vi "Begin.vi"(8 "error in":errorcluster) -> (0 "error out":errorcluster)   [LabVIEW 2016]
doc: "Called before other user functions, this VI is expected to open initial I/O refnums, load in file data, and do all program initialization. Notice that the <B>error out</B> terminal is simply used for data flow. Wiring it to other structures or subVIs ensures that this VI runs first."
uses:
  <vilib>/Rock Robotics/SystemInterfaces/DIO/FPGA_DIOPWMChannel.ctl
  <vilib>/Rock Robotics/WPI/SafetyOutput/WPI_SafetyOutputConfigMenu.ctl
  <vilib>/Rock Robotics/WPI/DriverStation/WPI_DriverStationRobotMode2.ctl
  <vilib>/Rock Robotics/WPI/Joystick/WPI_JoystickDeviceEnum.ctl
  <vilib>/Rock Robotics/SystemInterfaces/DIO/FPGA_DIOChannel.ctl
  <vilib>/Rock Robotics/WPI/RobotDrive/WPI_RobotDriveOpen2MotorWithVictorSP.vi
  Robot Global Data.vi
  <vilib>/Rock Robotics/Network Tables/NT Write String Array.vi
  <vilib>/Rock Robotics/WPI/MotorControl/WPI_MotorControlOpen SPARK.vi
  <vilib>/Rock Robotics/WPI/MotorControl/WPI_MotorControlOpen VictorSP.vi
  <vilib>/Rock Robotics/WPI/Counter/WPI_CounterDigitalInputToDigitalSource.vi
  <vilib>/Rock Robotics/WPI/Counter/WPI_CounterOpen UpDown Mode.vi
  <vilib>/Rock Robotics/WPI/Switch/WPI_SwitchOpenLimit.vi
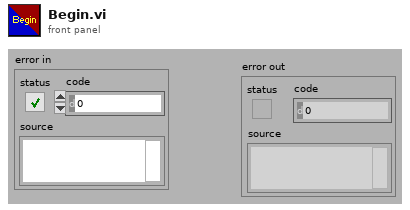
[diagram p1: front panel]
types:
  T1 = typedef "FPGA_DIOPWMChannel.ctl" = enum8{"PWM 0", "PWM 1", "PWM 2", "PWM 3", "PWM 4", "PWM 5", "PWM 6", "PWM 7", "PWM 8", "PWM 9", "PWM MXP 0", "PWM MXP 1", "PWM MXP 2", "PWM MXP 3", "PWM MXP 4", "PWM MXP 5", "PWM MXP 6", "PWM MXP 7", "PWM MXP 8", "PWM MXP 9", "Invalid"}
  T2 = typedef "FPGA_DIOChannel.ctl" = enum8{"DIO 0", "DIO 1", "DIO 2", "DIO 3", "DIO 4", "DIO 5", "DIO 6", "DIO 7", "DIO 8", "DIO 9", "DIO MXP 0", "DIO MXP 1", "DIO MXP 2", "DIO MXP 3", "DIO MXP 4", "DIO MXP 5", "DIO MXP 6", "DIO MXP 7", "DIO MXP 8", "DIO MXP 9", "DIO MXP 10", "DIO MXP 11", "DIO MXP 12", "DIO MXP 13", "DIO MXP 14", "DIO MXP 15", "SPI Port CS1", "SPI Port CS2", "SPI Port CS3", "SPI Port MISO", "SPI Port MOSI", "Invalid"}
  T3 = typedef "WPI_JoystickDeviceEnum.ctl" = enum16{"USB 0", "USB 1", "USB 2", "USB 3", "USB 4", "USB 5"}
  T4 = typedef "WPI_DriverStationRobotMode2.ctl" = enum16{"Autonomous Disabled", "Autonomous Enabled", "Teleop Disabled", "Teleop Enabled", "Disconnected", "Finish", "Test Disabled", "Test Enabled", "Emergency Stopped"}
  T5 = typedef "WPI_SafetyOutputConfigMenu.ctl" = enum16{"Enable", "Disable"}
  T6 = typedef "WPI_JoystickDevRef.ctl" = cluster{"Device":T3}
  T7 = typedef "WPI_SwitchDevRef.ctl" = cluster{"DevStatus":errorcluster, "DIO Channel":T2, "CntIndex":T8, "Normally Closed":bool}
  T8 = typedef "FPGA_CounterCtrSystemIndex.ctl" = enum8{"Ctr 0", "Ctr 1", "Ctr 2", "Ctr 3", "Ctr 4", "Ctr 5", "Ctr 6", "Ctr 7", "Invalid"}
  T9 = typedef "WPI_MotorControlDeviceRef.ctl" = cluster{"DeviceStatus":errorcluster, "Type":T10, "PWM":cluster{"PWM Channel":T1, "DeadBand":T11}, "CAN":cluster{"Device Number":u8, "SetOutput VI Ref":variant, "GetOutput VI Ref":variant, "Enable VI Ref":variant, "Disable VI Ref":variant, "Data":variant}, "Invert":bool}
  T10 = typedef "WPI_MotorControlType.ctl" = enum16{"PWM", "CAN"}
  T11 = typedef "WPI_PWMDeadband.ctl" = cluster{"Name":string, "maxPositivePwm":i32, "minPositivePwm":i32, "centerPwm":i32, "maxNegativePwm":i32, "minNegativePwm":i32, "angularRange":u16}
  T12 = typedef "WPI_RobotDriveDevRef.ctl" = cluster{"DevStatus":errorcluster, "Motors[]":T9[], "Square Inputs":bool, "Max Output":dbl}
  T13 = typedef "WPI_ServoDeviceRef.ctl" = cluster{"DeviceStatus":errorcluster, "PWM Channel":T1, "DeadBand":T11}
  T14 = typedef "WPI_DigitalInputDevRef.ctl" = cluster{"DevStatus":errorcluster, "DIO Channel":T2}
  T15 = typedef "FPGA_CounterEncoderSourceConvertionLVSourceType.ctl" = cluster{"DevStatus":errorcluster, "AnalogTriggerMode?":bool, "DigitalMode":cluster{"DIO Channel":T16}, "AnalogTriggerMode":cluster{"AnalogTriggerIndex":T17, "OutputType":T18}}
  T16 = typedef "FPGA_DIODigitalSourceChannel.ctl" = enum8{"DIO 0", "DIO 1", "DIO 2", "DIO 3", "DIO 4", "DIO 5", "DIO 6", "DIO 7", "DIO 8", "DIO 9", "DIO MXP 0", "DIO MXP 1", "DIO MXP 2", "DIO MXP 3", "DIO MXP 4", "DIO MXP 5", "DIO MXP 6", "DIO MXP 7", "DIO MXP 8", "DIO MXP 9", "DIO MXP 10", "DIO MXP 11", "DIO MXP 12", "DIO MXP 13", "DIO MXP 14", "DIO MXP 15", "Disabled"}
  T17 = typedef "FPGA_AnalogTriggerIndex.ctl" = enum8{"Trig 0", "Trig 1", "Trig 2", "Trig 3", "Trig 4", "Trig 5", "Trig 6", "Trig 7", "Invalid"}
  T18 = typedef "FPGA_AnalogTriggerOutType.ctl" = enum16{"InWindow", "TriggerState", "Rising", "Falling"}
  T19 = typedef "WPI_CounterDevRef.ctl" = cluster{"DevStatus":errorcluster, "CntIndex":T8}
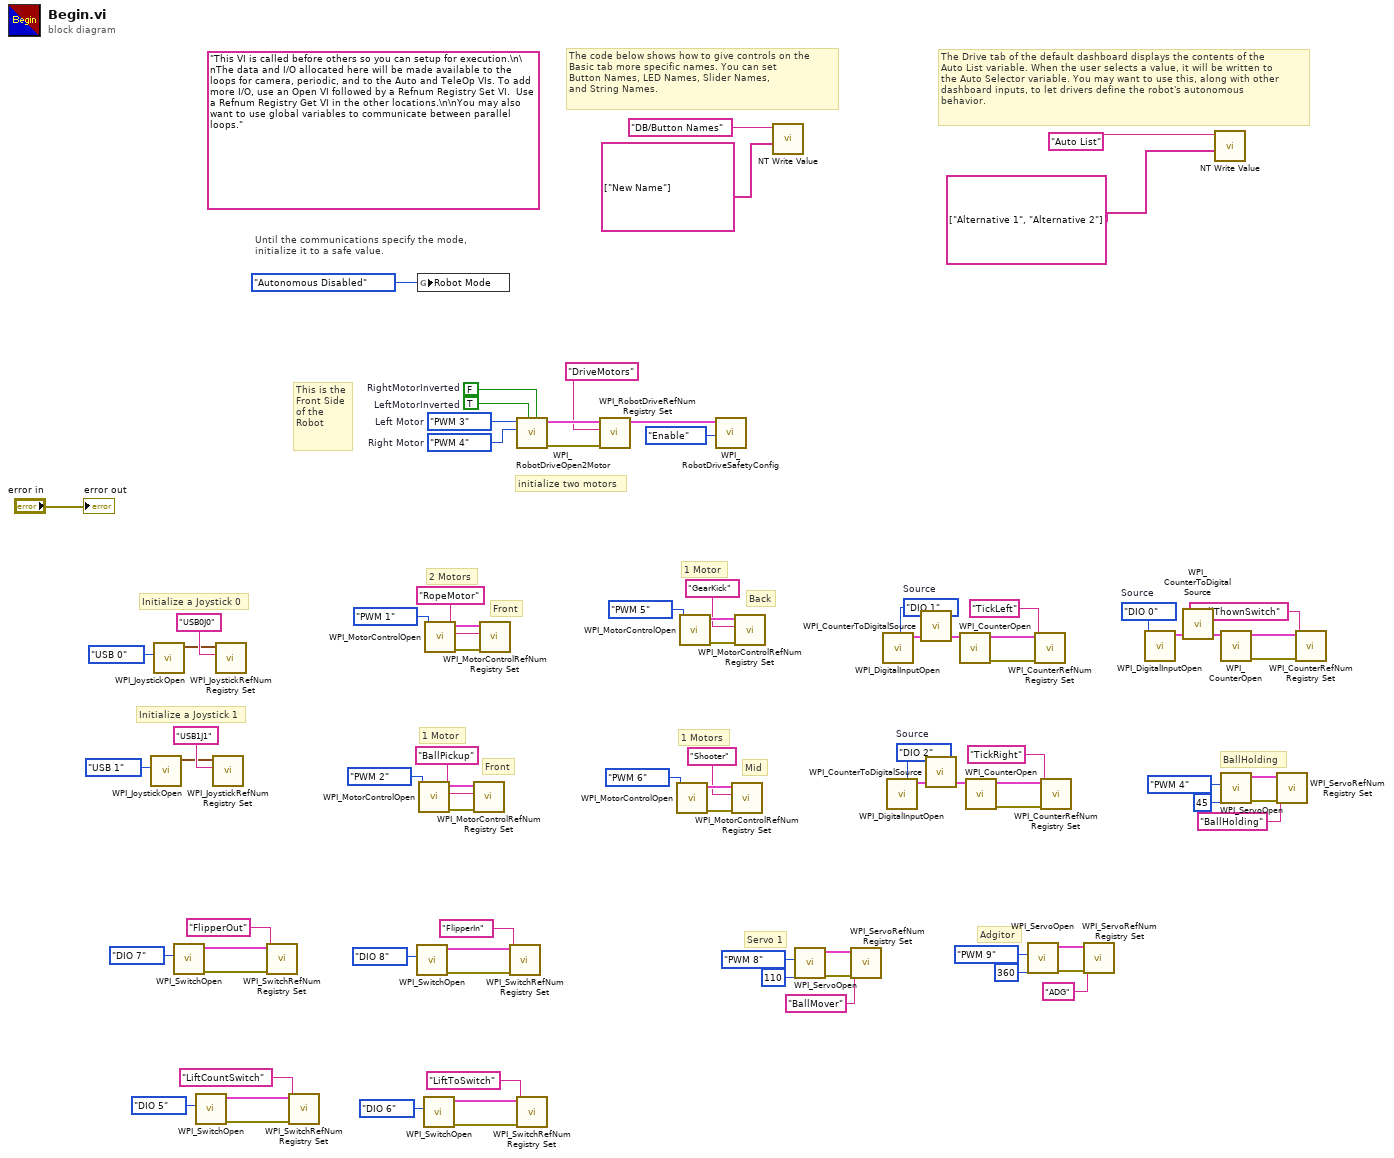
[diagram p0: block diagram]
diagram:
  w36 = FPGA_DIOChannel."DIO 0"  # Source
  w42 = FPGA_DIOChannel."DIO 2"  # Source
  w48 = FPGA_DIOChannel."DIO 1"  # Source
  (unwired) "This VI is called before others so you can setup for execution.\n\nThe data and I/O allocated here will be made available to the loops for camera, periodic, and to the Auto and TeleOp VIs. To add more I/O, use an Open VI followed by a Refnum Registry Set VI.  Use a Refnum Registry Get VI in the other locations.\n\nYou may also want to use global variables to communicate between parallel loops."
  w80 = FPGA_DIOPWMChannel."PWM 4"  # Right Motor
  w81 = FPGA_DIOPWMChannel."PWM 3"  # Left Motor
  w85 = TRUE  # LeftMotorInverted
  w86 = FALSE  # RightMotorInverted
  # "Adgitor"
  # "Servo 1"
  # "BallHolding"
  # "Mid"
  # "Back"
  # "Front"
  # "Front"
  # "This is the Front Side of the Robot"
  # "1 Motors"
  # "1 Motor"
  # "1 Motor"
  # "2 Motors"
  # "Initialize a Joystick 1"
  # "The Drive tab of the default dashboard displays the contents of the\nAuto List variable. When the user selects a value, it will be written to\nthe Auto Selector variable. You may want to use this, along with other\ndashboard inputs, to let drivers define the robot's autonomous\nbehavior."
  # "The code below shows how to give controls on the\nBasic tab more specific names. You can set\nButton Names, LED Names, Slider Names,\nand String Names."
  # "Initialize a Joystick 0"
  # "Until the communications specify the mode,\ninitialize it to a safe value."
  # "initialize two motors"
  n1 = call <vilib>:"WPI_JoystickOpen.vi"("JoystickDevice"=WPI_JoystickDeviceEnum."USB 1") -> ("JoystickDevRef"=w67:T6)  [unwired: 10 in]
  n2 = call <vilib>:"WPI_JoystickOpen.vi"("JoystickDevice"=WPI_JoystickDeviceEnum."USB 0") -> ("JoystickDevRef"=w75:T6)  [unwired: 10 in]
  n3 = call-poly <vilib>:"WPI_SwitchOpen.vi"("DIO Channel"=FPGA_DIOChannel."DIO 7") -> ("error out"=w26:errorcluster, "SwitchDevRef"=w25:T7)  [unwired: 9 in]
  n4 = call-poly <vilib>:"WPI_SwitchOpen.vi"("DIO Channel"=FPGA_DIOChannel."DIO 5") -> ("error out"=w18:errorcluster, "SwitchDevRef"=w17:T7)  [unwired: 9 in]
  n5 = call <vilib>:"WPI_JoystickRefNum Registry Set.vi"("refnum name"="USB1J1", "JoystickDevRef"=w67) -> ()  [unwired: 8 in, 2 out]
  n6 = call <vilib>:"WPI_JoystickRefNum Registry Set.vi"("refnum name"="USB0J0", "JoystickDevRef"=w75) -> ()  [unwired: 8 in, 2 out]
  n7 = call <vilib>:"WPI_SwitchRefNum Registry Set.vi"("error in (no error)"=w26, "refnum name"="FlipperOut", "SwitchDevRef"=w25) -> ()  [unwired: 7 in, 2 out]
  n8 = call <vilib>:"WPI_SwitchRefNum Registry Set.vi"("error in (no error)"=w18, "refnum name"="LiftCountSwitch", "SwitchDevRef"=w17) -> ()  [unwired: 7 in, 2 out]
  n9 = call-poly <vilib>:"WPI_SwitchOpen.vi"("DIO Channel"=FPGA_DIOChannel."DIO 8") -> ("error out"=w22:errorcluster, "SwitchDevRef"=w21:T7)  [unwired: 9 in]
  n10 = global write "Robot Global Data.vi" "Robot Mode"(WPI_DriverStationRobotMode2."Autonomous Disabled" ("Robot Mode")) -> ()
  n11 = call-poly <vilib>:"WPI_MotorControlOpen.vi"("PWM Channel"=FPGA_DIOPWMChannel."PWM 2") -> ("error out"=w65:errorcluster, "MotorControlDeviceRef"=w64:T9)  [unwired: 9 in]
  n12 = call-poly <vilib>:"WPI_SwitchOpen.vi"("DIO Channel"=FPGA_DIOChannel."DIO 6") -> ("error out"=w14:errorcluster, "SwitchDevRef"=w13:T7)  [unwired: 9 in]
  n13 = call-poly <vilib>:"WPI_MotorControlOpen.vi"("PWM Channel"=FPGA_DIOPWMChannel."PWM 1") -> ("error out"=w61:errorcluster, "MotorControlDeviceRef"=w60:T9)  [unwired: 9 in]
  n14 = call <vilib>:"WPI_MotorControlRefNum Registry Set.vi"("error in (no error)"=w65, "refnum name"="BallPickup", "MotorControlDevRef"=w64) -> ()  [unwired: 7 in, 2 out]
  n15 = call <vilib>:"WPI_MotorControlRefNum Registry Set.vi"("error in (no error)"=w61, "refnum name"="RopeMotor", "MotorControlDevRef"=w60) -> ()  [unwired: 7 in, 2 out]
  n16 = call <vilib>:"WPI_SwitchRefNum Registry Set.vi"("error in (no error)"=w22, "refnum name"="FlipperIn", "SwitchDevRef"=w21) -> ()  [unwired: 7 in, 2 out]
  n17 = call-poly <vilib>:"WPI_RobotDriveOpen2Motor.vi"("Right Motor Inverted"=w86, "Left Motor Inverted"=w85, "Right Motor"=w80, "Left Motor"=w81) -> ("error out"=w82:errorcluster, "RobotDriveDevRef"=w84:T12)  [unwired: 1 in, 5 out]
  n18 = call <vilib>:"WPI_SwitchRefNum Registry Set.vi"("error in (no error)"=w14, "refnum name"="LiftToSwitch", "SwitchDevRef"=w13) -> ()  [unwired: 7 in, 2 out]
  n19 = call <vilib>:"WPI_RobotDriveRefNum Registry Set.vi"("error in (no error)"=w82, "refnum name"="DriveMotors", "RobotDriveDevRef"=w84) -> ("RobotDriveDevRef"=w79:T12)  [unwired: 1 in, 7 out]
  n20 = call-poly <vilib>:"WPI_MotorControlOpen.vi"("PWM Channel"=FPGA_DIOPWMChannel."PWM 6") -> ("error out"=w53:errorcluster, "MotorControlDeviceRef"=w52:T9)  [unwired: 9 in]
  n21 = call-poly <vilib>:"WPI_MotorControlOpen.vi"("PWM Channel"=FPGA_DIOPWMChannel."PWM 5") -> ("error out"=w57:errorcluster, "MotorControlDeviceRef"=w56:T9)  [unwired: 9 in]
  n22 = call <vilib>:"WPI_RobotDriveSafetyConfig.vi"("mode"=WPI_SafetyOutputConfigMenu."Enable", "RobotDriveDevRef"=w79) -> ()  [unwired: 8 in, 2 out]
  n23 = call <vilib>:"WPI_MotorControlRefNum Registry Set.vi"("error in (no error)"=w53, "refnum name"="Shooter", "MotorControlDevRef"=w52) -> ()  [unwired: 7 in, 2 out]
  n24 = call <vilib>:"WPI_MotorControlRefNum Registry Set.vi"("error in (no error)"=w57, "refnum name"="GearKick", "MotorControlDevRef"=w56) -> ()  [unwired: 7 in, 2 out]
  n25 = call-poly <vilib>:"NT Write Value.vi"("String Array"=string[] ["New Name"], "Name"="DB/Button Names") -> ()  [unwired: 9 in, 1 out]
  n26 = call <vilib>:"WPI_ServoOpen.vi"("Angular Range"=u16 110, "PWM Channel"=FPGA_DIOPWMChannel."PWM 8") -> ("error out"=w8:errorcluster, "ServoDeviceRef"=w7:T13)  [unwired: 8 in]
  n27 = call <vilib>:"WPI_ServoRefNum Registry Set.vi"("error in (no error)"=w8, "refnum name"="BallMover", "ServoDeviceRef"=w7) -> ()  [unwired: 7 in, 2 out]
  n28 = call <vilib>:"WPI_DigitalInputOpen.vi"("DIO Channel"=w48) -> ("DigitalInputDevRef"=w47:T14)  [unwired: 1 in, 9 out]
  n29 = call <vilib>:"WPI_DigitalInputOpen.vi"("DIO Channel"=w42) -> ("DigitalInputDevRef"=w41:T14)  [unwired: 1 in, 9 out]
  n30 = call-poly <vilib>:"WPI_CounterToDigitalSource.vi"("DigitalInputDevRef"=w47) -> ("Digital Source"=w49:T15)  [unwired: 6 out]
  n31 = call-poly <vilib>:"WPI_CounterToDigitalSource.vi"("DigitalInputDevRef"=w41) -> ("Digital Source"=w43:T15)  [unwired: 6 out]
  n32 = call-poly <vilib>:"WPI_CounterOpen.vi"("Up Source"=w49) -> ("error out"=w46:errorcluster, "CounterDevRef"=w45:T19)  [unwired: 6 in, 3 out]
  n33 = call-poly <vilib>:"WPI_CounterOpen.vi"("Up Source"=w43) -> ("error out"=w40:errorcluster, "CounterDevRef"=w39:T19)  [unwired: 6 in, 3 out]
  n34 = call <vilib>:"WPI_ServoOpen.vi"("Angular Range"=u16 360, "PWM Channel"=FPGA_DIOPWMChannel."PWM 9") -> ("error out"=w3:errorcluster, "ServoDeviceRef"=w2:T13)  [unwired: 8 in]
  n35 = call <vilib>:"WPI_CounterRefNum Registry Set.vi"("error in (no error)"=w46, "refnum name"="TickLeft", "CounterDevRef"=w45) -> ()  [unwired: 7 in, 2 out]
  n36 = call <vilib>:"WPI_CounterRefNum Registry Set.vi"("error in (no error)"=w40, "refnum name"="TickRight", "CounterDevRef"=w39) -> ()  [unwired: 7 in, 2 out]
  n37 = call <vilib>:"WPI_ServoRefNum Registry Set.vi"("error in (no error)"=w3, "refnum name"="ADG", "ServoDeviceRef"=w2) -> ()  [unwired: 7 in, 2 out]
  n38 = call <vilib>:"WPI_DigitalInputOpen.vi"("DIO Channel"=w36) -> ("DigitalInputDevRef"=w35:T14)  [unwired: 1 in, 9 out]
  n39 = call-poly <vilib>:"WPI_CounterToDigitalSource.vi"("DigitalInputDevRef"=w35) -> ("Digital Source"=w37:T15)  [unwired: 6 out]
  n40 = call-poly <vilib>:"NT Write Value.vi"("String Array"=string[] ["Alternative 1", "Alternative 2"], "Name"="Auto List") -> ()  [unwired: 9 in, 1 out]
  n41 = call-poly <vilib>:"WPI_CounterOpen.vi"("Up Source"=w37) -> ("error out"=w34:errorcluster, "CounterDevRef"=w33:T19)  [unwired: 6 in, 3 out]
  n42 = call <vilib>:"WPI_ServoOpen.vi"("Angular Range"=u16 45, "PWM Channel"=FPGA_DIOPWMChannel."PWM 4") -> ("error out"=w29:errorcluster, "ServoDeviceRef"=w28:T13)  [unwired: 8 in]
  n43 = call <vilib>:"WPI_ServoRefNum Registry Set.vi"("error in (no error)"=w29, "refnum name"="BallHolding", "ServoDeviceRef"=w28) -> ()  [unwired: 7 in, 2 out]
  n44 = call <vilib>:"WPI_CounterRefNum Registry Set.vi"("error in (no error)"=w34, "refnum name"="BallThownSwitch", "CounterDevRef"=w33) -> ()  [unwired: 7 in, 2 out]
  "error out" <- "error in"
